vi "get ID from vi.vi"(11 "VI in":refnum<vi>) -> (2 "owning library":string, 3 "VI ID":string)   [LabVIEW 2020]
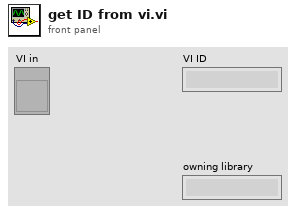
[diagram p1: front panel]
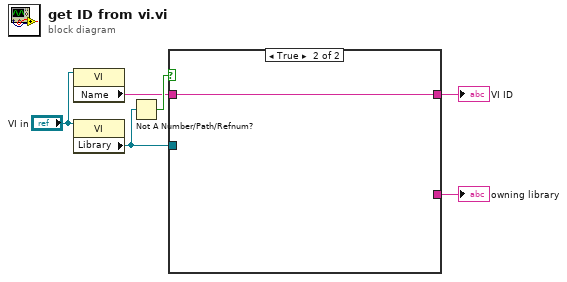
[diagram p0: block diagram]
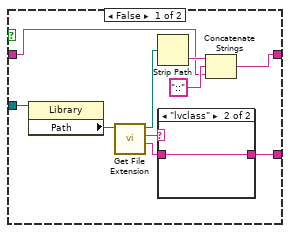
[diagram p2: hidden frame]
diagram:
  n1 = property class="VI"(reference="VI in") -> ("Name"=w1:string)  [unwired: 1 in, 2 out]
  n2 = property class="VI"(reference="VI in") -> ("Library"=w4:refnum<vi>)  [unwired: 1 in, 2 out]
  n3 = Not A Number/Path/Refnum?(number/path/refnum=w4) -> (NaN/Path/Refnum?=w5:bool)
  n4 = case shown="True" w5 {
    tunnel: w4 -> [w16 _]
    tunnel: [w12 _] -> w3
    tunnel: w1 -> [w8 w18]
    tunnel: [w7 w18] -> w6
    frame False {
      n5 = property class="Library"(reference=w16) -> ("Path"=w15:path)  [unwired: 1 in, 2 out]
      n6 = call <vilib>:"Get File Extension.vi"("file"=w15) -> ("filename without extension"=w13:string, "lowercase file extension"=w14:string, "dup file"=w11:path)  [unwired: 6 in, 2 out]
      n7 = Strip Path(path=w11) -> (name=w10:string)  [unwired: 1 out]
      n8 = case shown="\"lvclass\"" w14 {
        tunnel: w13 -> [_ w17]
        tunnel: [_ w17] -> w12
        frame Default {
        }
        frame "lvclass" {
        }
      }
      n9 = Concatenate Strings(w10, "::" ("string"), w8) -> (w7:string)
    }
    frame True {
    }
  }
  "VI ID" <- w6
  "owning library" <- w3
